vi "Linear Scaling with Points.vi"(1 "Point2":cluster{"x2":dbl, "y2":dbl}, 2 "Point1":cluster{"x1":dbl, "y1":dbl}, 3 "Input":dbl) -> (0 "Output":dbl)   [LabVIEW 2021]
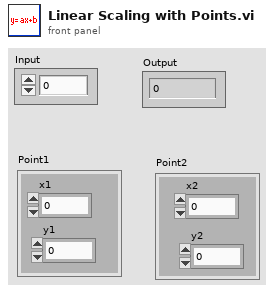
[diagram p1: front panel]
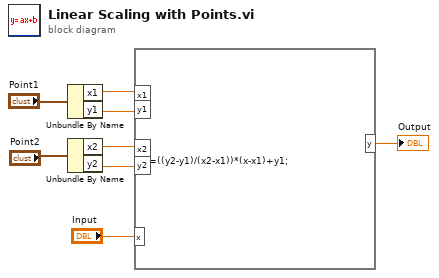
[diagram p0: block diagram]
diagram:
  n1 = Unbundle By Name("Point1") -> ("x1"=w4:dbl, "y1"=w3:dbl)
  n2 = Unbundle By Name("Point2") -> ("x2"=w2:dbl, "y2"=w1:dbl)
  n3 = formula code="y=((y2-y1)/(x2-x1))*(x-x1)+y1;"("x1"=w4, "y1"=w3, "x2"=w2, "y2"=w1, "x"="Input") -> ("y"=→"Output":dbl)
